vi "Root Element.vi"(8 "error in (no error)":errorcluster, 10 "Config":refnum<class "Config Manager.lvclass">, 11 "Config Storage in":refnum<class "Config Storage.lvclass">) -> (0 "error out":errorcluster, 2 "Root":refnum<class "Config Element.lvclass">, 3 "Config Storage out":refnum<class "Config Storage.lvclass">, 5 "Subtree Added":bool)   [LabVIEW 2020, in "CDM-Config.lvlib" / "Config Storage.lvclass"]
uses:
  Config Storage.lvclass
  Config Manager/Config Manager.lvclass
  Config Element/Config Element.lvclass
  Config Storage.lvclass/Config Storage.ctl
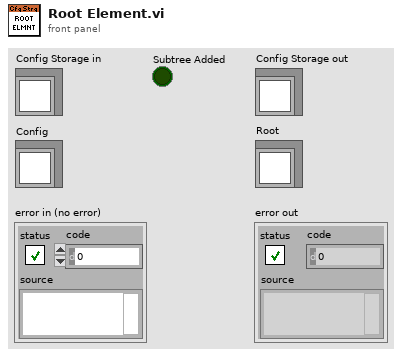
[diagram p1: front panel]
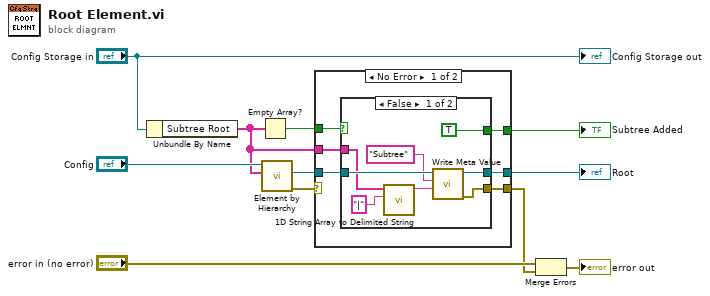
[diagram p0: block diagram]
diagram:
  n1 = Unbundle By Name("Config Storage in") -> ("Subtree Root"=w6:string[])
  n2 = Empty Array?(array=w6) -> (empty?=w7:bool)
  n3 = call "Element by Hierarchy.vi"("Hierarchy"=w6, "Config Manager in"="Config") -> ("error out"=w3:errorcluster, "Config Element"=w8:refnum<class "Config Element.lvclass">)  [unwired: 7 in, 1 out]
  n4 = case shown="No Error" w3 {
    selector: w3 -> [_ w27]
    tunnel: w8 -> [w17 _]
    tunnel: w7 -> [w16 _]
    tunnel: w6 -> [w15 _]
    tunnel: [w14 _] -> w5
    tunnel: [w13 _] -> w4
    tunnel: [w12 w27] -> w1
    frame No Error {
      n5 = case shown="False" w16 {
        tunnel: w17 -> [w25 w26]
        tunnel: w15 -> [w21 _]
        tunnel: [w23 w26] -> w14
        tunnel: [TRUE _] -> w13
        tunnel: [w18 _] -> w12
        frame False {
          n6 = call <vilib>:"1D String Array to Delimited String.vi"("delimiter"="|", "string array"=w21) -> ("delimited string"=w19:string)  [unwired: 9 in]
          n7 = call "Write Meta Value.vi"("Meta Value"=w19, "Meta Name"="Subtree", "Config Element in"=w25) -> ("error out"=w18:errorcluster, "Config Element out"=w23:refnum<class "Config Element.lvclass">)  [unwired: 7 in]
        }
        frame True {
        }
      }
    }
    frame Error {
    }
  }
  "Root" <- w5
  "Subtree Added" <- w4
  n8 = Merge Errors("error in (no error)", w1) -> (→"error out":errorcluster)
  "Config Storage out" <- "Config Storage in"
